vi "PV VOC Data.vi"(11 "result string":string) -> (3 "Boolean":bool)   [LabVIEW 2023]
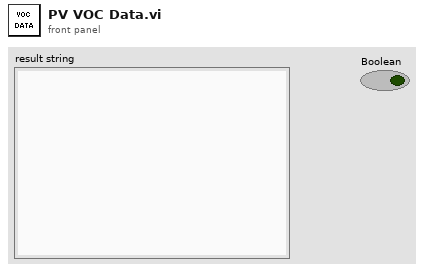
[diagram p1: front panel]
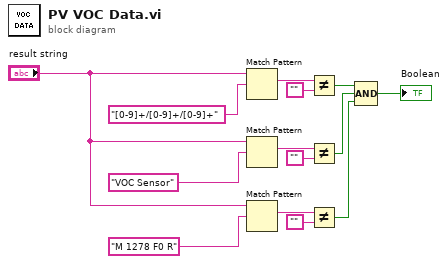
[diagram p0: block diagram]
diagram:
  n1 = Match Pattern(string="result string", regular expression="[0-9]+/[0-9]+/[0-9]+" ("string")) -> (match substring=w7:string)  [unwired: 1 in, 3 out]
  n2 = Match Pattern(string="result string", regular expression="VOC Sensor" ("string")) -> (match substring=w2:string)  [unwired: 1 in, 3 out]
  n3 = Match Pattern(string="result string", regular expression="M 1278 F0 R" ("string")) -> (match substring=w5:string)  [unwired: 1 in, 3 out]
  n4 = Not Equal?(x=w7, y="") -> (x != y?=w10:bool)
  n5 = Not Equal?(x=w2, y="") -> (x != y?=w11:bool)
  n6 = Not Equal?(x=w5, y="") -> (x != y?=w12:bool)
  n7 = Compound Arithmetic op=AND(w10, w11, w12) -> (→"Boolean":bool)
